vi "Make Writable - VI.vi"(8 "error in (no error)":errorcluster, 11 "VI in":refnum<vi>) -> (0 "error out":errorcluster, 3 "VI out":refnum<vi>)   [LabVIEW 2015, in "UniquifyFullyQualifiedVIName.lvclass"]
uses:
  UniquifyFullyQualifiedVIName.lvclass
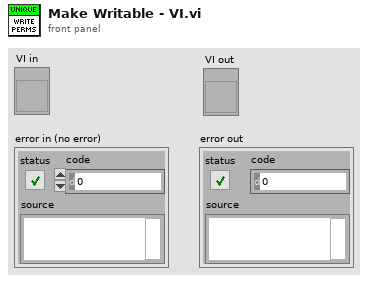
[diagram p1: front panel]
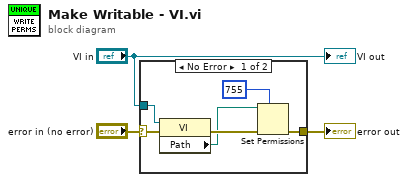
[diagram p0: block diagram]
diagram:
  n1 = case shown="No Error" "error in (no error)" {
    selector: "error in (no error)" -> [w7 w10]
    tunnel: [w6 w10] -> w2
    tunnel: "VI in" -> [w4 _]
    frame No Error {
      n2 = property class="VI"(reference=w4, error in=w7) -> (error out=w9:errorcluster, "Path"=w5:path)  [unwired: 1 out]
      n3 = Set Permissions(7:i16 755 ("permissions"), 8:w9, 11:w5) -> (0:w6:errorcluster)  [unwired: 2 in, 1 out]
    }
    frame Error {
    }
  }
  "error out" <- w2
  "VI out" <- "VI in"
